vi "System@TimerCheck__Parameter.vi"(1 "ParamterIn":string) -> (0 "ParamterOut":string)   [LabVIEW 2020]
panel:
  in  "Timer":string(combo)
  in  "Confirm":bool
  # "System@TimerCheck $Timer"
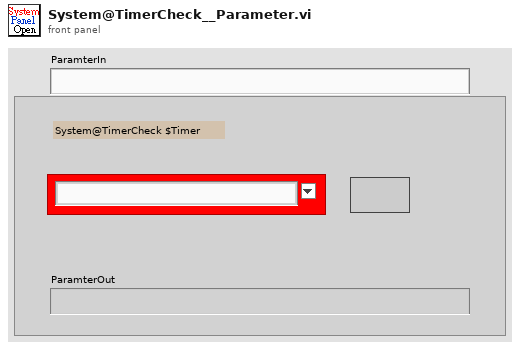
[diagram p1: front panel]
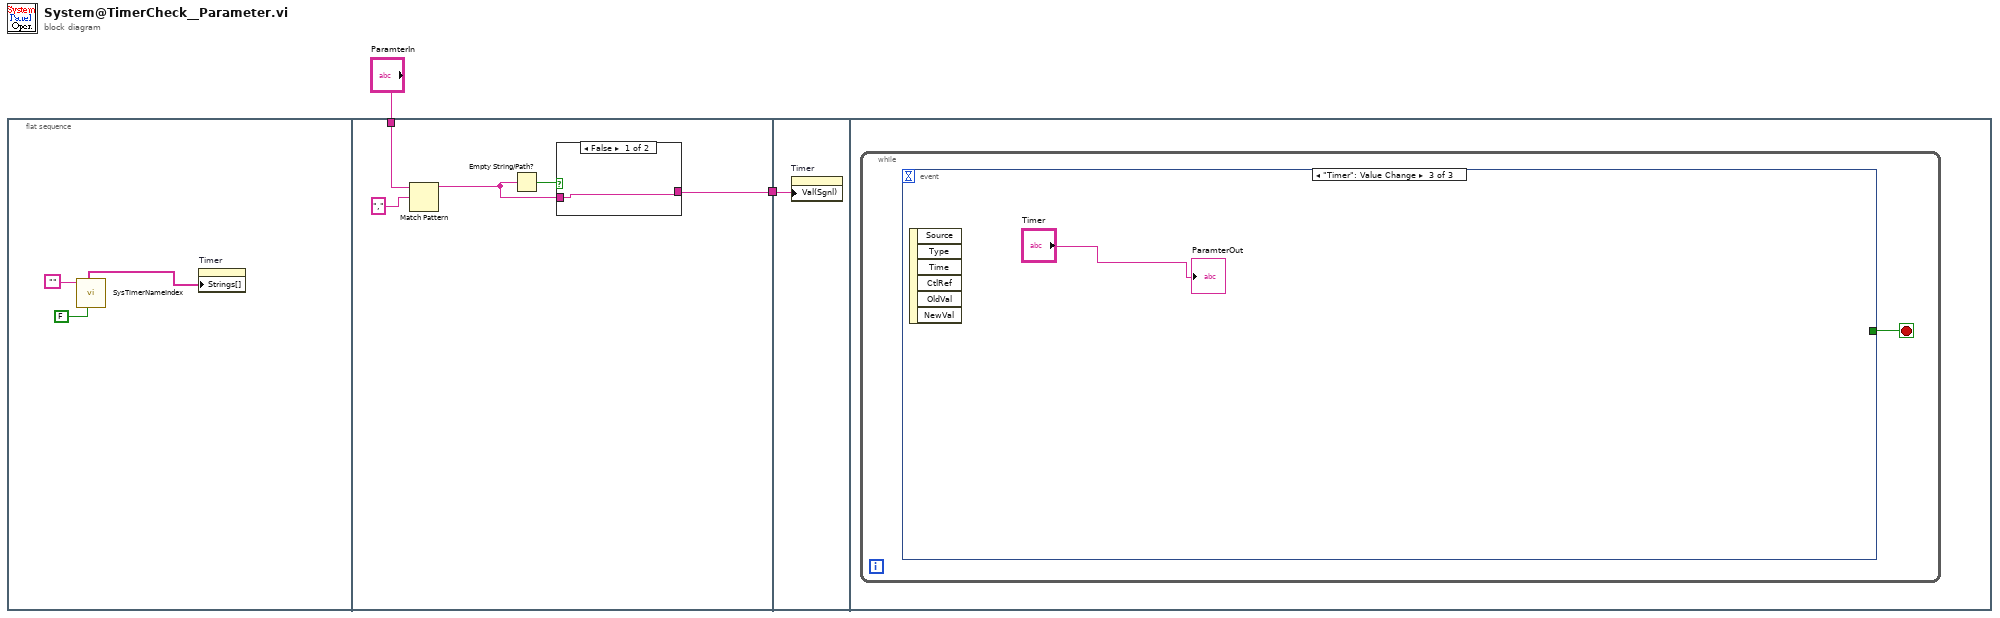
[diagram p0: block diagram]
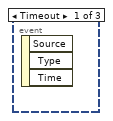
[diagram p3: hidden frame]
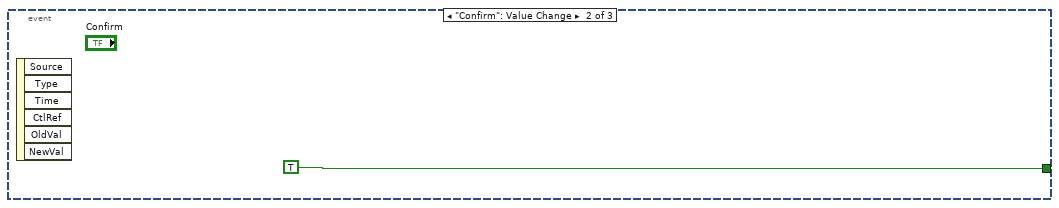
[diagram p4: hidden frame]
diagram:
  n1 = flat-sequence {
    tunnel: "ParamterIn" -> [w9]
    tunnel: [w6] -> w1
    tunnel: w1 -> [w13]
    frame #0 {
      n2 = call "SysTimerNameIndex.vi"("Reset"=FALSE, "TimerName"="") -> ("NameList"=w3:string[])  [unwired: 7 in, 2 out]
      n3 = property on="Timer" class="CmbBox"("Strings[]"=w3) -> ()  [unwired: 2 in, 2 out]
    }
    frame #1 {
      n4 = Match Pattern(string=w9, regular expression=",") -> (before substring=w7:string)  [unwired: 1 in, 3 out]
      n5 = Empty String/Path?(string/path=w7) -> (empty?=w10:bool)
      n6 = case shown="False" w10 {
        tunnel: w7 -> [w11 w12]
        tunnel: [w11 w12] -> w6
        frame False {
        }
        frame True {
        }
      }
    }
    frame #2 {
      n7 = property on="Timer" class="CmbBox"("Val(Sgnl)"=w13) -> ()  [unwired: 2 in, 2 out]
    }
    frame #3 {
      n8 = while {
        stop <- w14 stop-if-true
        n9 = event shown="[2] \"Timer\": Value Change" {
          selector: _ -> [_ _ _]
          dyn-events: _ -> [_ _ _]
          timeout: _ -> [_ _ _]
          tunnel: [_ TRUE _] -> w14
          event Timeout {
            n10 = event-data() -> ()  [unwired: 1 in, 3 out]
          }
          event "Confirm": Value Change {
            n11 = event-data() -> ()  [unwired: 1 in, 6 out]
          }
          event "Timer": Value Change {
            n12 = event-data() -> ()  [unwired: 1 in, 6 out]
            "ParamterOut" <- "Timer"
          }
        }
      }
    }
  }
